vi "UWB_Controller.vi"() -> ()   [LabVIEW 2016]
doc: "This VI controlls the DWM over UART. It starts of by resetting the DWM by sending a reset message over UART. It then starts sending CR messages to the DWM and poll for a response. When anything is received on the poll the DWM is operational. It then starts to request a position message which it saves in a global variable later used by the ROS publisher."
uses:
  <vilib>/myRIO/Instrument Drivers/Onboard IO/AO/typedefs/AO Reference.ctl
  <vilib>/myRIO/Common/Instrument Driver Framework/Utilities/typedefs/myRIO Generic Hardware Reference.ctl
  <vilib>/myRIO/Common/Instrument Driver Framework/Utilities/typedefs/Hardware Version Enum.ctl
  <vilib>/myRIO/Common/Instrument Driver Framework/Utilities/typedefs/myRIO v1.0 Reference.ctl
  <vilib>/myRIO/Common/Instrument Driver Framework/Utilities/typedefs/Generic FPGA Reference.ctl
  <vilib>/myRIO/Common/Instrument Driver Framework/myRIO v1.0/AO/typedefs/AO Channels List.ctl
  <vilib>/myRIO/Common/Instrument Driver Framework/myRIO v1.0/AO/typedefs/AO Channels Enum.ctl
  <vilib>/myRIO/Common/Instrument Driver Framework/Utilities/typedefs/Analog Scaling Constants List.ctl
  <vilib>/myRIO/Common/Instrument Driver Framework/Utilities/typedefs/Analog Scaling Constants.ctl
  <vilib>/userdefined/High Color/nirio_resource_hc.ctl
  <vilib>/myRIO/Instrument Drivers/Onboard IO/UART/typedef/VISA Configuration.ctl
  <vilib>/myRIO/Instrument Drivers/Onboard IO/DIO/typedefs/DIO Reference.ctl
  <vilib>/myRIO/Common/Instrument Driver Framework/myRIO v1.0/DIO/typedefs/DIO Channels List.ctl
  <vilib>/myRIO/Common/Instrument Driver Framework/myRIO v1.0/DIO/typedefs/DIO Channels Enum.ctl
  <vilib>/myRIO/Common/Instrument Driver Framework/Utilities/vis/Is FPGA Ref Available.vi
  <vilib>/myRIO/Common/Instrument Driver Framework/roboRIO v1.0/AO/vis/roboRIO v1.0 Open AO.vi
  <vilib>/myRIO/Instrument Drivers/Onboard IO/AO/vis/Write.vi
  <vilib>/myRIO/Common/Instrument Driver Framework/roboRIO v1.0/DIO/vis/roboRIO v1.0 Open DIO.vi
  <vilib>/myRIO/Instrument Drivers/Onboard IO/DIO/vis/Write.vi
  <vilib>/myRIO/Common/Instrument Driver Framework/Utilities/vis/Validate Channels.vi
  <vilib>/myRIO/Common/Instrument Driver Framework/roboRIO v1.0/AO/vis/roboRIO v1.0 Reserve AO.vi
  <vilib>/myRIO/Common/Instrument Driver Framework/roboRIO v1.0/DIO/vis/roboRIO v1.0 Reserve DIO.vi
  <vilib>/myRIO/Common/Instrument Driver Framework/roboRIO v1.0/AO/vis/roboRIO v1.0 Build MUX Configuration AO.vi
  <vilib>/myRIO/Common/Instrument Driver Framework/roboRIO v1.0/Resource Manager/vis/roboRIO v1.0 Reserve Channel List.vi
  <vilib>/myRIO/Common/Instrument Driver Framework/roboRIO v1.0/DIO/vis/roboRIO v1.0 Build MUX Configuration DIO.vi
  <vilib>/myRIO/Common/Instrument Driver Framework/roboRIO v1.0/Resource Manager/vis/roboRIO v1.0 Reserve Channel.vi
  <vilib>/myRIO/Common/Instrument Driver Framework/roboRIO v1.0/Resource Manager/vis/roboRIO v1.0 Unreserve Channel.vi
  <vilib>/myRIO/Common/Instrument Driver Framework/roboRIO v1.0/Resource Manager/vis/roboRIO v1.0 Create Configuration List.vi
  <vilib>/myRIO/Common/Instrument Driver Framework/roboRIO v1.0/Resource Manager/vis/roboRIO v1.0 Build Mutex Name.vi
  <vilib>/Instr/_visa.llb/VISA Configure Serial Port (Instr).vi
  GlobalVI.vi
  <vilib>/Utility/VariantDataType/GetNumericInfo.vi
  <vilib>/Utility/error.llb/Error Cluster From Error Code.vi
  <vilib>/myRIO/Common/Instrument Driver Framework/roboRIO v1.0/roboRIO v1.0 Open.vi
  <vilib>/myRIO/Common/Instrument Driver Framework/Utilities/vis/IO Manager.vi
  <vilib>/myRIO/Common/Instrument Driver Framework/Utilities/vis/Configuration Manager.vi
  <vilib>/myRIO/Common/Instrument Driver Framework/roboRIO v1.0/Resource Manager/vis/roboRIO v1.0 Configure IO.vi
  <vilib>/myRIO/Common/Instrument Driver Framework/myRIO v1.0/myRIO v1.0 Close.vi
  <vilib>/myRIO/Common/Instrument Driver Framework/roboRIO v1.0/DIO/vis/roboRIO v1.0 Write DIO.vi
  <vilib>/myRIO/Common/Instrument Driver Framework/roboRIO v1.0/AO/vis/roboRIO v1.0 Get Scaling Constants AO.vi
  <vilib>/myRIO/Common/Instrument Driver Framework/roboRIO v1.0/AO/vis/roboRIO v1.0 Write AO.vi
  <vilib>/myRIO/Express VI/Onboard IO/UART/UART Express VI.xnode
  <vilib>/regexp/Match Regular Expression.xnode
  <vilib>/myRIO/Express VI/Onboard Devices/LED/LED Express VI.xnode
  <vilib>/myRIO/Instrument Drivers/Onboard IO/DIO/vis/myRIO DIO Open.xnode
  <vilib>/myRIO/Express VI/Onboard IO/AO/AO Express VI.xnode
  <vilib>/myRIO/Instrument Drivers/Onboard IO/AO/vis/myRIO AO Open.xnode
  <vilib>/myRIO/Instrument Drivers/Onboard IO/UART/UART.lvlib
  <vilib>/myRIO/Instrument Drivers/Onboard IO/DIO/DIO.lvlib
  <vilib>/myRIO/Instrument Drivers/Onboard IO/AO/AO.lvlib
panel:
  in  "error in OUTPUT 3":errorcluster
  in  "error in INPUT 2":errorcluster
  out "currentTimeout_Receive":u32
  out "error out OUTPUT 2":errorcluster
  out "offset past match\n(-1 = no match)":i32
  out "MSGFound":bool
  out "X":dbl
  out "Y":dbl
  out "Z":dbl
  out "error out INPUT":errorcluster
  out "timeoutError":bool
  out "currentTimeout":u32
  out "timeoutCount":u32
  out "timeoutValue":u32
  out "Resetting...":bool
  out "System ON":bool
  out "Receiving":bool
  out "Transmitting":bool
  out "UART Reset Buffer":string
  out "uwbState":i32
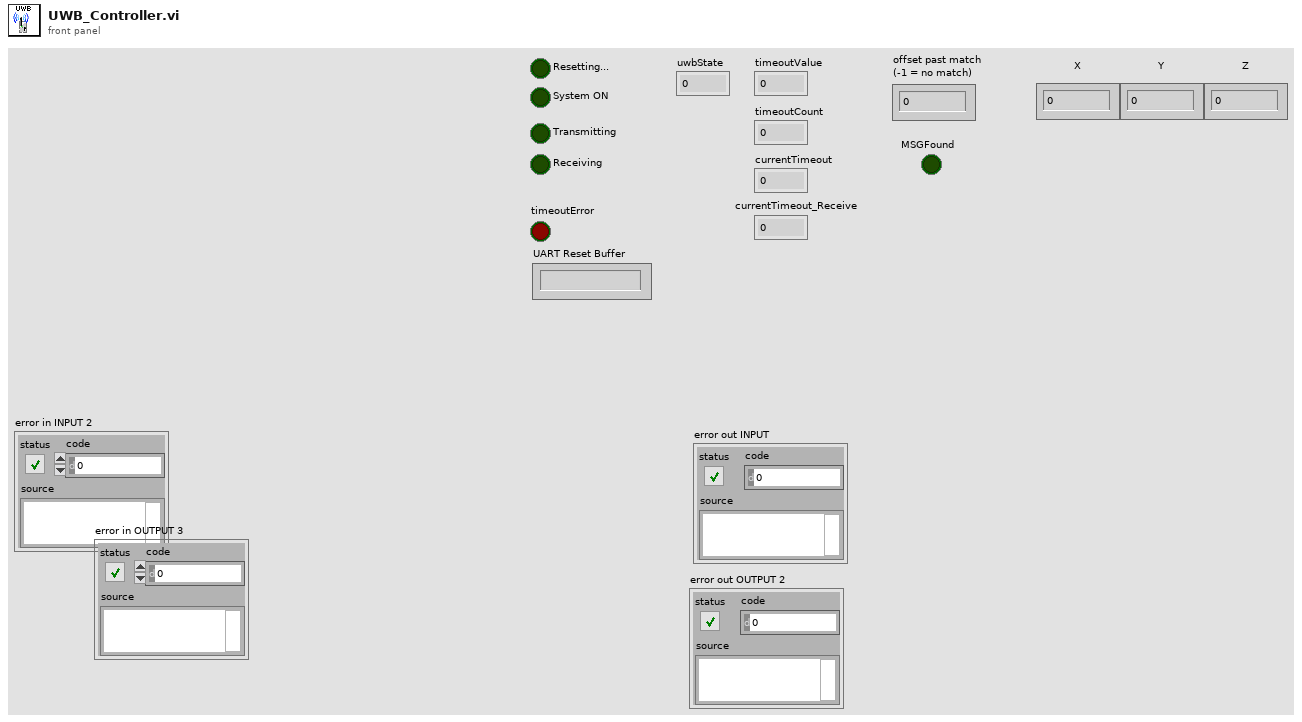
[diagram p1: front panel]
types:
  T1 = typedef "UART.lvlib/VISA Configuration.ctl" = cluster{"baud rate (9600)":u32, "data bits (8)":u16, "parity (0:none)":enum16{"None", "Odd", "Even", "Mark", "Space"}, "stop bits (10: 1 bit)":u16, "flow control (0:none)":u16, "termination char\n(0xA = '\\n' = LF) ":u8, "Enable Termination\nChar (T)":bool, "timeout (10sec)":u32}
  T2 = typedef "DIO.lvlib/DIO Reference.ctl" = cluster{"myRIO Reference":T3, "DIO Channels List":T7}
  T3 = typedef "myRIO Generic Hardware Reference.ctl" = cluster{"myRIO Model":T4, "myRIO Hardware Reference":T5}
  T4 = typedef "Hardware Version Enum.ctl" = enum16{"Unknown", "myRIO-1900", "myRIO-1950", "roboRIO", "NI ELVIS RIO CM"}
  T5 = typedef "myRIO v1.0 Reference.ctl" = cluster{"Generic FPGA Reference":T6, "Allow multiple opens":bool}
  T6 = typedef "Generic FPGA Reference.ctl" = refnum<k20>
  T7 = typedef "DIO Channels List.ctl" = T8[]
  T8 = typedef "DIO Channels Enum.ctl" = enum16{"Not Connected", "C/DIO0", "C/DIO1", "C/DIO2", "C/DIO3", "C/DIO4", "C/DIO5", "C/DIO6", "C/DIO7", "A/DIO0", "A/DIO1", "A/DIO2", "A/DIO3", "A/DIO4", "A/DIO5", "A/DIO6", "A/DIO7", "A/DIO8", "A/DIO9", "A/DIO10", "A/DIO11", "A/DIO12", "A/DIO13", "A/DIO14", "A/DIO15", "B/DIO0", "B/DIO1", "B/DIO2", "B/DIO3", "B/DIO4", "B/DIO5", "B/DIO6", "B/DIO7", "B/DIO8", "B/DIO9", "B/DIO10", "B/DIO11", "B/DIO12", "B/DIO13", "B/DIO14", "B/DIO15", "LED0", "LED1", "LED2", "LED3", "Button0", "DIO/DIO0", "DIO/DIO1", "DIO/DIO2", "DIO/DIO3", "DIO/DIO4", "DIO/DIO5", "DIO/DIO6", "DIO/DIO7", "DIO/DIO8", "DIO/DIO9", "SPI/CS0", "SPI/CS1", "SPI/CS2", "SPI/CS3", "LED RADIO (Green)", "LED RADIO (Red)", "LED COMM (Green)", "LED COMM (Red)", "LED MODE (Green)", "LED MODE (Red)"}
  T9 = typedef "nirio_resource_hc.ctl" = tag
  T10 = typedef "AO.lvlib/AO Reference.ctl" = cluster{"myRIO Reference":T3, "AO Channel List":T11, "AO Scaling Constant List":T13}
  T11 = typedef "AO Channels List.ctl" = T12[]
  T12 = typedef "AO Channels Enum.ctl" = enum16{"Not Connected", "AudioOut/Left", "AudioOut/Right", "C/AO0", "C/AO1", "A/AO0", "A/AO1", "B/AO0", "B/AO1"}
  T13 = typedef "Analog Scaling Constants List.ctl" = T14[]
  T14 = typedef "Analog Scaling Constants.ctl" = cluster{"LSB Weight (Volts)":dbl, "Offset (Volts)":dbl, "Signed?":bool}
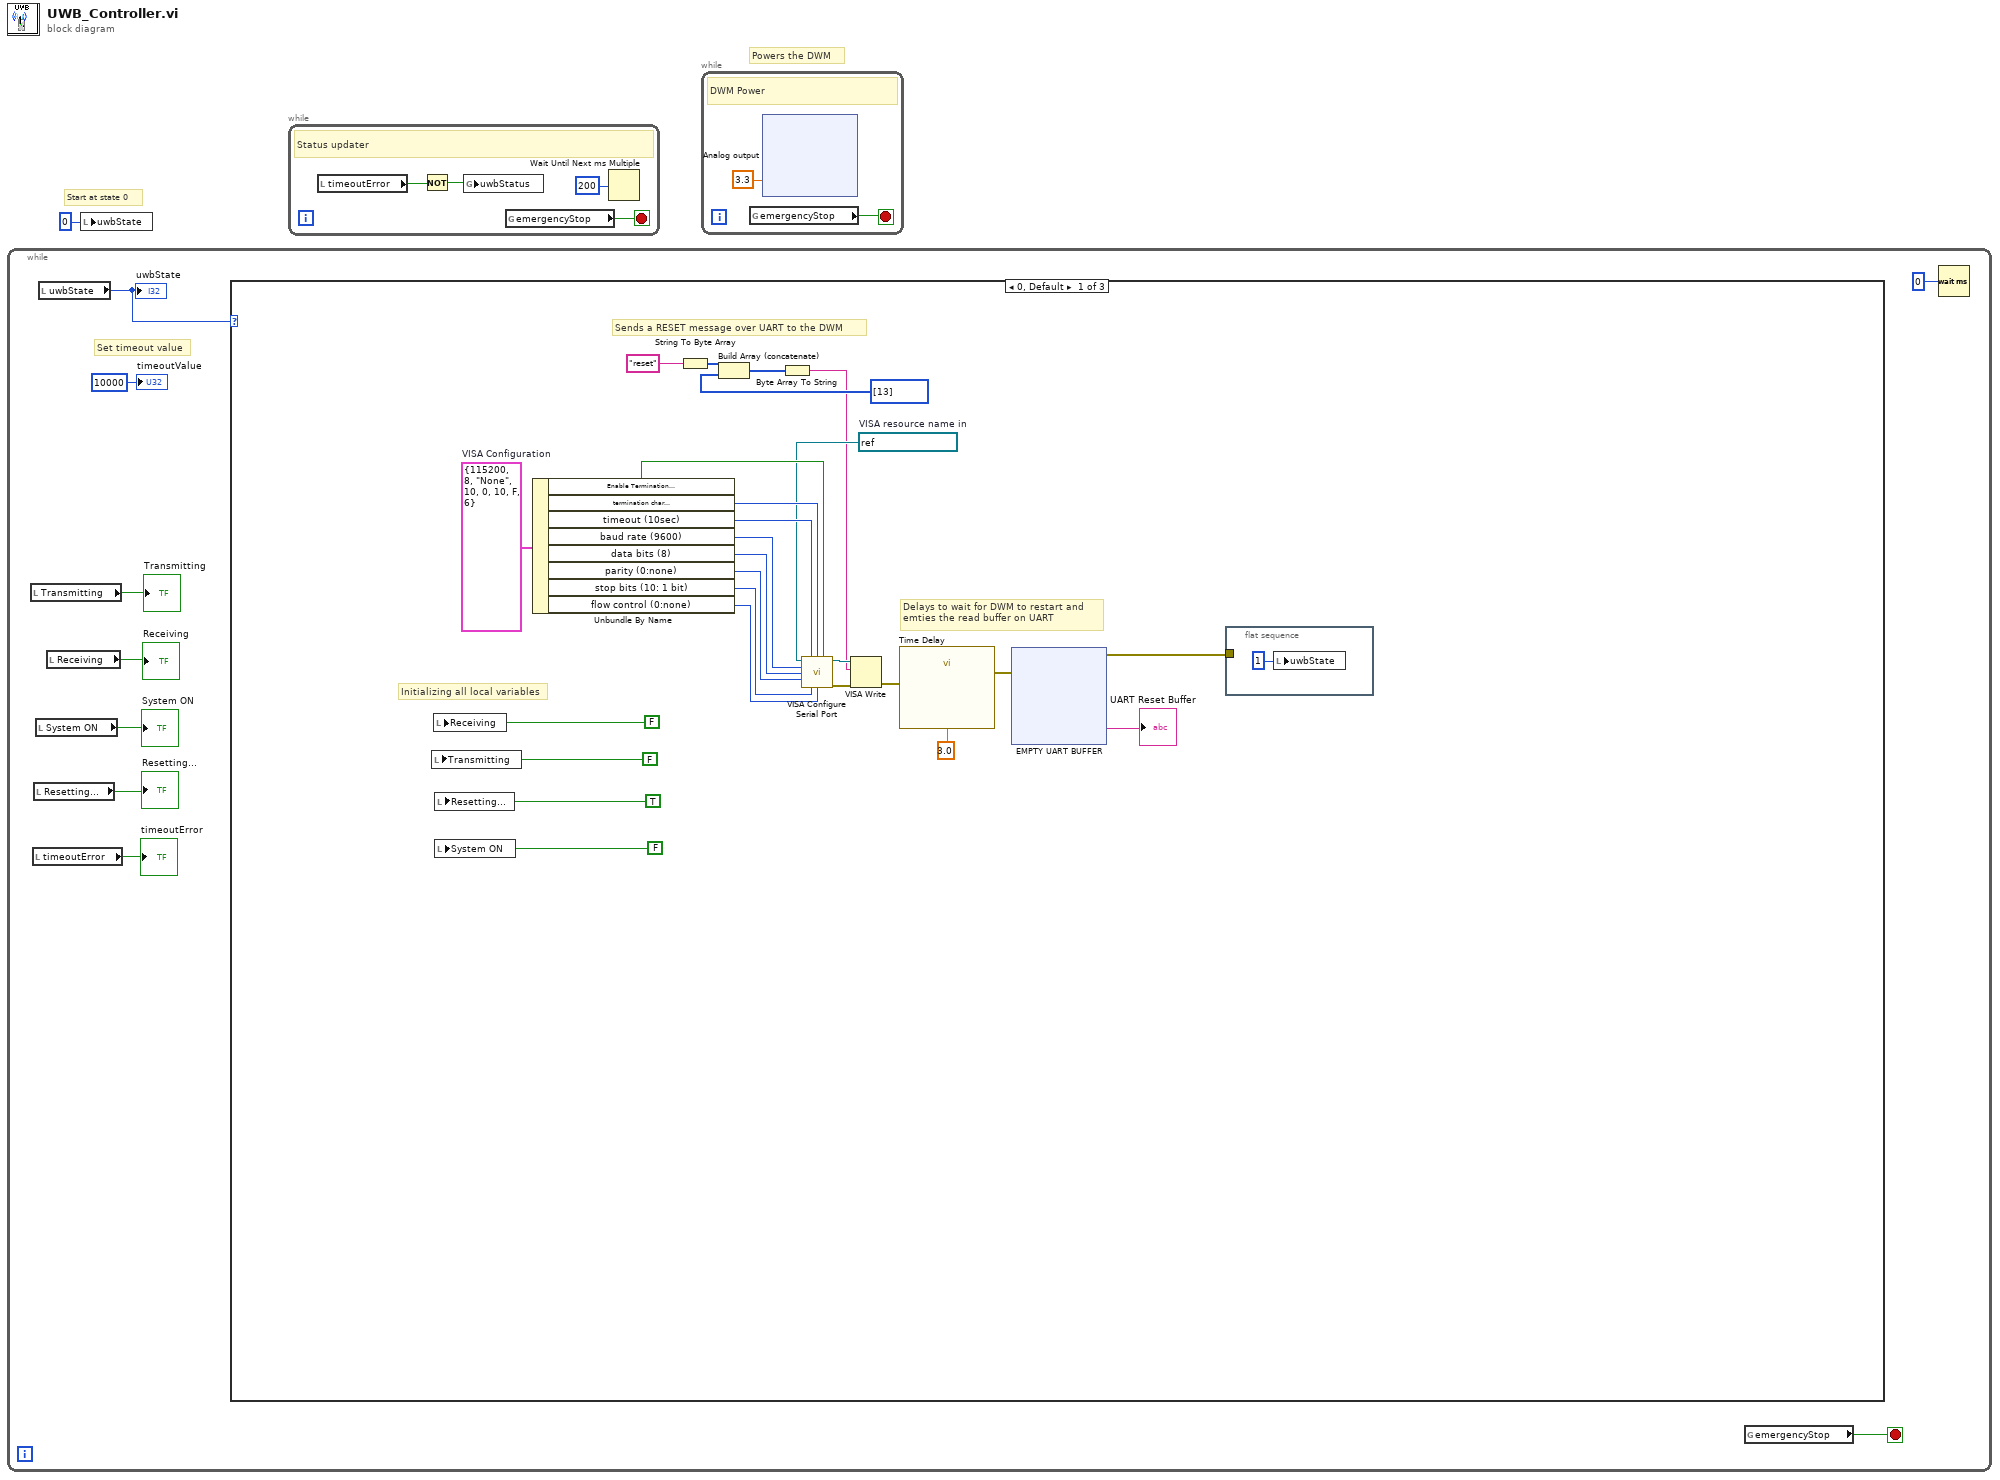
[diagram p0: block diagram]
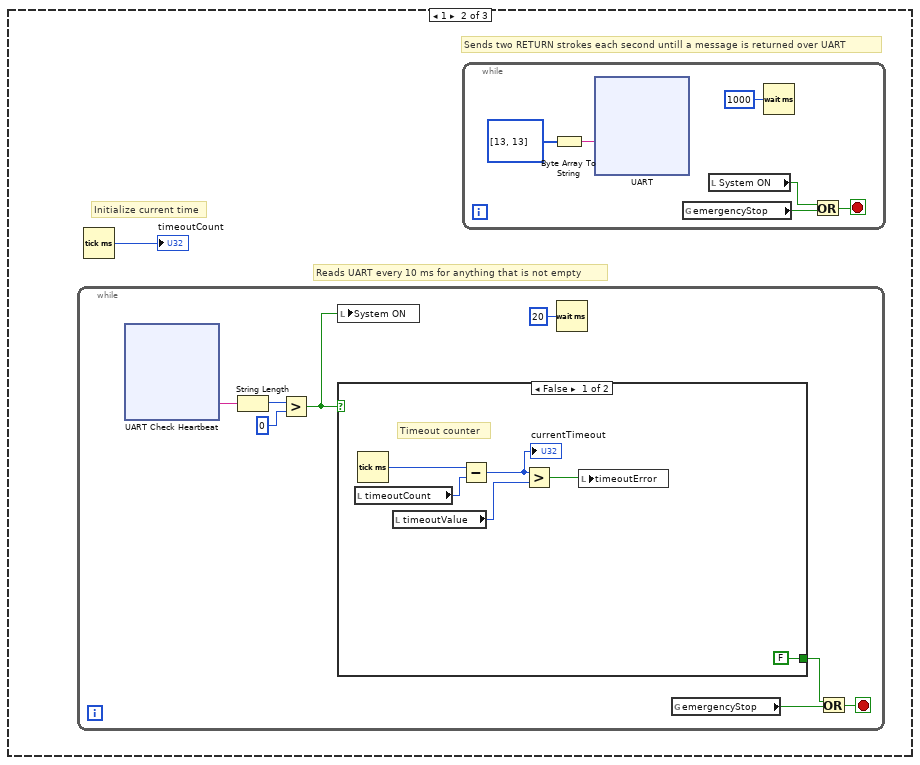
[diagram p2: hidden frame]
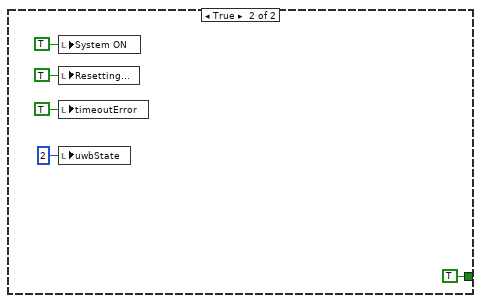
[diagram p3: hidden frame]
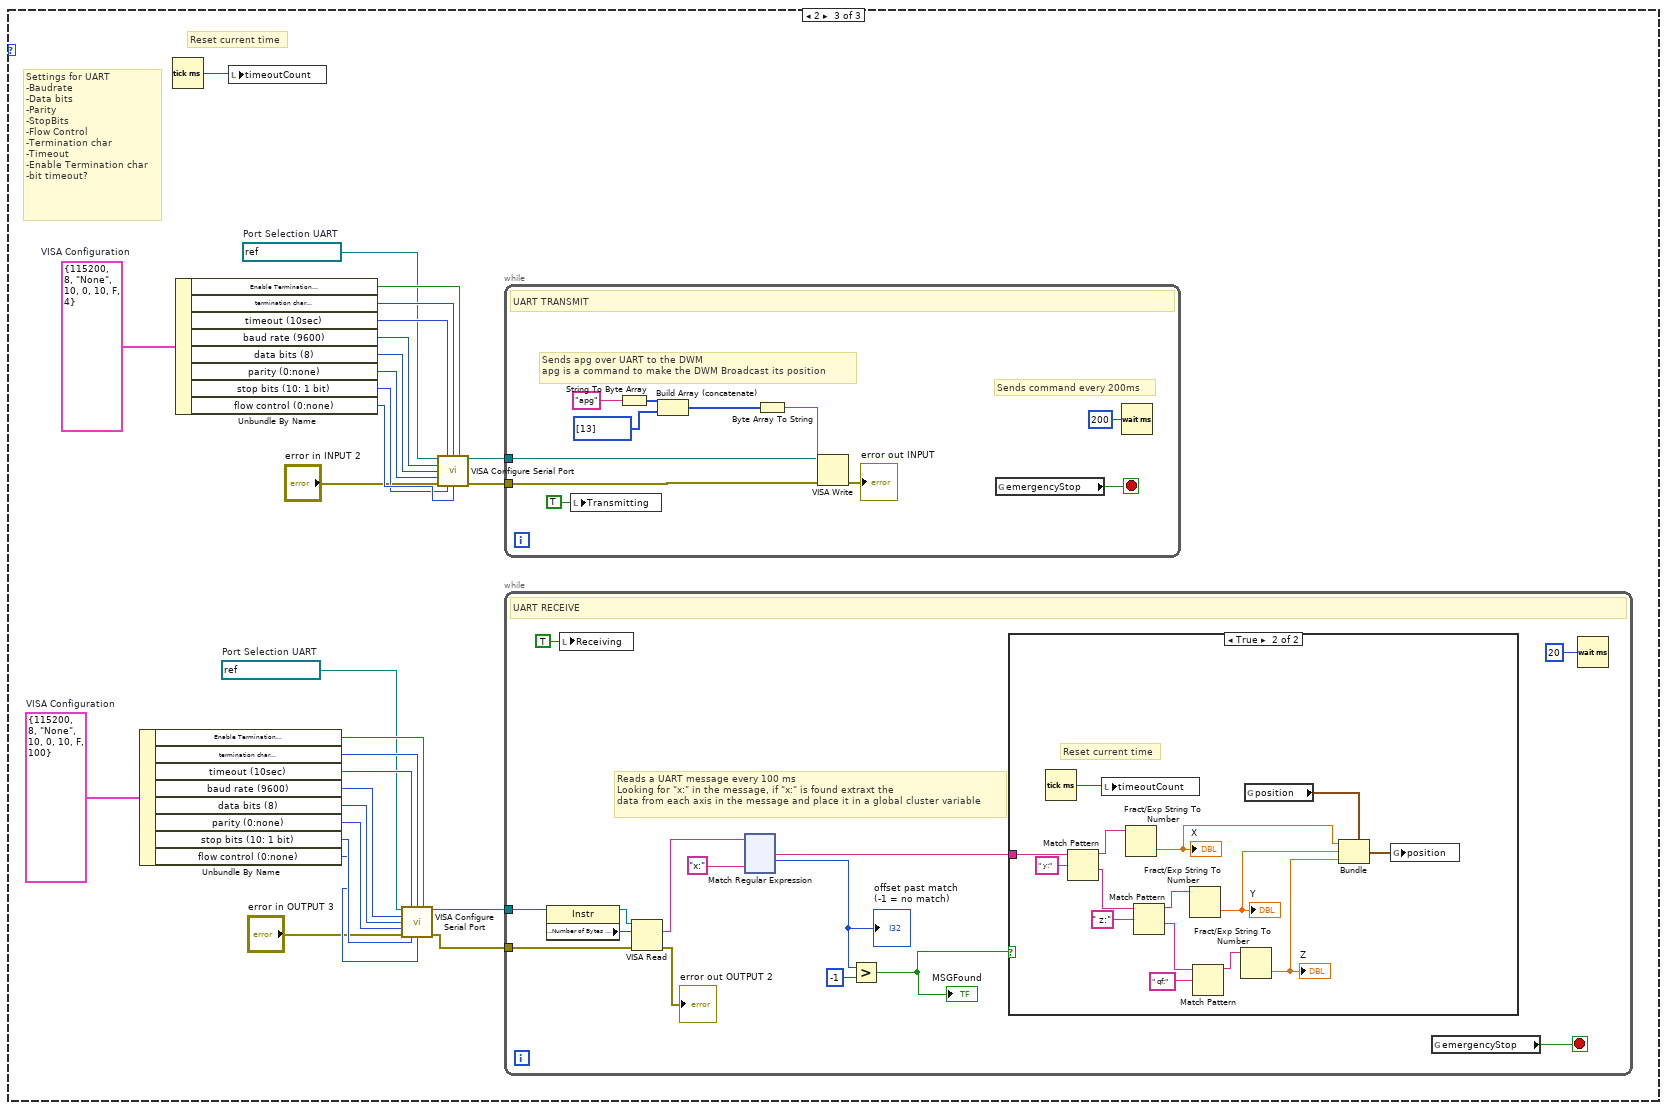
[diagram p4: hidden frame]
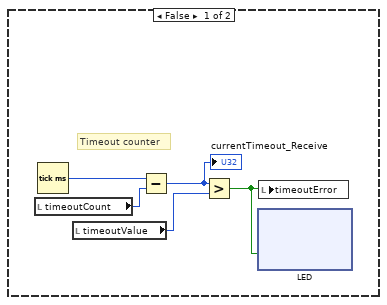
[diagram p5: hidden frame]
diagram:
  # "Powers the DWM"
  # "Start at state 0"
  n1 = while {
    stop <- w6 stop-if-true
    # "Set timeout value"
    n2 = local read "Transmitting"() -> (→"Transmitting":bool)
    n3 = local read "timeoutError"() -> (→"timeoutError":bool)
    n4 = local read "Resetting..."() -> (→"Resetting...":bool)
    n5 = local read "System ON"() -> (→"System ON":bool)
    n6 = local read "uwbState"() -> (w4:i32)
    "uwbState" <- w4
    n7 = local read "Receiving"() -> (→"Receiving":bool)
    n8 = case shown="0, Default" w4 {
      frame 0, Default {
        w24 = T1 {"baud rate (9600)"=115200, "data bits (8)"=8, "parity (0:none)"=enum."None", "stop bits (10: 1 bit)"=10, "flow control (0:none)"=0, "termination char\n(0xA = '\\n' = LF) "=10, "Enable Termination\nChar (T)"=FALSE, "timeout (10sec)"=6}  # VISA Configuration
        w23 = refnum<visa-resource-name> "ASRL2::INSTR"  # VISA resource name in
        # "Initializing all local variables"
        # "Delays to wait for DWM to restart and \nemties the read buffer on UART"
        # "Sends a RESET message over UART to the DWM"
        n9 = local write "Transmitting"(FALSE ("Transmitting")) -> ()
        n10 = local write "Receiving"(FALSE ("Receiving")) -> ()
        n11 = local write "Resetting..."(TRUE ("Resetting...")) -> ()
        n12 = local write "System ON"(FALSE ("System On")) -> ()
        n13 = Unbundle By Name(w24) -> ("Enable Termination\nChar (T)"=w27:bool, "termination char\n(0xA = '\\n' = LF)"=w28:u8, "timeout (10sec)"=w29:u32, "baud rate (9600)"=w34:u32, "data bits (8)"=w33:u16, "parity (0:none)"=w32:enum16{"None", "Odd", "Even", "Mark", "Space"}, "stop bits (10: 1 bit)"=w31:u16, "flow control (0:none)"=w30:u16)
        n14 = String To Byte Array(string="reset") -> (unsigned byte array=w19:u8[])
        n15 = Build Array (concatenate)(w19, i32[] [13]) -> (w18:i32[])
        n16 = Byte Array To String(unsigned byte array=w18) -> (string=w17:string)
        n17 = call-poly "VISA Configure Serial Port"("VISA resource name"=w23, "timeout (10sec)"=w29, "termination char\n(0xA = '\\n' = LF)"=w28, "Enable Termination\nChar (T)"=w27, "baud rate (9600)"=w34, "data bits (8)"=w33, "parity (0:none)"=w32, "stop bits (10: 1 bit)"=w31, "flow control (0:none)"=w30) -> ("VISA resource name out"=w25:refnum<visa-resource-name>, "error out"=w26:errorcluster)  [unwired: 5 in]
        n18 = VISA Write(VISA resource name=w25, write buffer=w17, error in (no error)=w26) -> (error out=w22:errorcluster)  [unwired: 2 out]
        n19 = call "Time Delay"("error in (no error)"=w22, "Delay Time (s)"=3.0) -> ("error out"=w35:errorcluster)  [unwired: 9 in]
        n20 = xnode "EMPTY UART BUFFER"("error in (no error)"=w35) -> ("Characters Read"=→"UART Reset Buffer":string, "error out"=w11:errorcluster)
        n21 = flat-sequence {
          tunnel: w11 -> [_]
          frame #0 {
            n22 = local write "uwbState"(1 ("uwbState")) -> ()
          }
        }
      }
      frame 1 {
        # "Initialize current time"
        # "Reads UART every 10 ms for anything that is not empty"
        # "Sends two RETURN strokes each second untill a message is returned over UART"
        n23 = while {
          stop <- w80 stop-if-true
          n24 = xnode "UART Check Heartbeat"() -> ("Characters Read"=w85:string)  [unwired: 1 in, 1 out]
          n25 = String Length(string=w85) -> (length=w84:i32)
          n26 = Greater?(x=w84, y=0) -> (0:w81:bool)
          n27 = local write "System ON"(w81) -> ()
          n28 = case shown="False" w81 {
            tunnel: [FALSE TRUE] -> w79
            frame False {
              # "Timeout counter"
              n29 = local read "timeoutCount"() -> (w88:u32)
              n30 = Tick Count (ms)() -> (millisecond timer value=w90:u32)
              n31 = local read "timeoutValue"() -> (w89:u32)
              n32 = Subtract(x=w90, y=w88) -> (x-y=w87:u32)
              "currentTimeout" <- w87
              n33 = Greater?(x=w87, y=w89) -> (0:w86:bool)
              n34 = local write "timeoutError"(w86) -> ()
            }
            frame True {
              n35 = local write "System ON"(TRUE ("System ON")) -> ()
              n36 = local write "Resetting..."(TRUE ("Resetting...")) -> ()
              n37 = local write "timeoutError"(TRUE ("timeoutError")) -> ()
              n38 = local write "uwbState"(2 ("uwbState")) -> ()
            }
          }
          n39 = Wait (ms)(milliseconds to wait=u32 20) -> ()  [unwired: 1 out]
          n40 = global read "GlobalVI.vi" "emergencyStop"() -> (w78:bool)
          n41 = Or(x=w79, y=w78) -> (x .or. y?=w80:bool)
        }
        n42 = Tick Count (ms)() -> (millisecond timer value=→"timeoutCount":u32)
        n43 = while {
          stop <- w57 stop-if-true
          n44 = Byte Array To String(unsigned byte array=u8[] [13, 13]) -> (string=w61:string)
          n45 = xnode "UART"("Characters to Write"=w61) -> ()  [unwired: 1 in, 2 out]
          n46 = global read "GlobalVI.vi" "emergencyStop"() -> (w58:bool)
          n47 = local read "System ON"() -> (w56:bool)
          n48 = Wait (ms)(milliseconds to wait=u32 1000) -> ()  [unwired: 1 out]
          n49 = Or(x=w56, y=w58) -> (x .or. y?=w57:bool)
        }
      }
      frame 2 {
        w117 = T1 {"baud rate (9600)"=115200, "data bits (8)"=8, "parity (0:none)"=enum."None", "stop bits (10: 1 bit)"=10, "flow control (0:none)"=0, "termination char\n(0xA = '\\n' = LF) "=10, "Enable Termination\nChar (T)"=FALSE, "timeout (10sec)"=100}  # VISA Configuration
        w116 = refnum<visa-resource-name> "ASRL2::INSTR"  # Port Selection UART
        w130 = T1 {"baud rate (9600)"=115200, "data bits (8)"=8, "parity (0:none)"=enum."None", "stop bits (10: 1 bit)"=10, "flow control (0:none)"=0, "termination char\n(0xA = '\\n' = LF) "=10, "Enable Termination\nChar (T)"=FALSE, "timeout (10sec)"=4}  # VISA Configuration
        w129 = refnum<visa-resource-name> "ASRL2::INSTR"  # Port Selection UART
        # "Settings for UART\n-Baudrate\n-Data bits\n-Parity\n-StopBits\n-Flow Control\n-Termination char\n-Timeout\n-Enable Termination char\n-bit timeout?"
        # "Reset current time"
        n50 = Unbundle By Name(w117) -> ("Enable Termination\nChar (T)"=w119:bool, "termination char\n(0xA = '\\n' = LF)"=w120:u8, "timeout (10sec)"=w121:u32, "baud rate (9600)"=w126:u32, "data bits (8)"=w125:u16, "parity (0:none)"=w124:enum16{"None", "Odd", "Even", "Mark", "Space"}, "stop bits (10: 1 bit)"=w123:u16, "flow control (0:none)"=w122:u16)
        n51 = Tick Count (ms)() -> (millisecond timer value=w140:u32)
        n52 = Unbundle By Name(w130) -> ("Enable Termination\nChar (T)"=w132:bool, "termination char\n(0xA = '\\n' = LF)"=w133:u8, "timeout (10sec)"=w134:u32, "baud rate (9600)"=w138:u32, "data bits (8)"=w137:u16, "parity (0:none)"=w136:enum16{"None", "Odd", "Even", "Mark", "Space"}, "stop bits (10: 1 bit)"=w135:u16, "flow control (0:none)"=w139:u16)
        n53 = local write "timeoutCount"(w140) -> ()
        n54 = call-poly "VISA Configure Serial Port"("VISA resource name"=w116, "timeout (10sec)"=w121, "termination char\n(0xA = '\\n' = LF)"=w120, "Enable Termination\nChar (T)"=w119, "baud rate (9600)"=w126, "data bits (8)"=w125, "parity (0:none)"=w124, "error in (no error)"="error in OUTPUT 3", "stop bits (10: 1 bit)"=w123, "flow control (0:none)"=w122) -> ("VISA resource name out"=w115:refnum<visa-resource-name>, "error out"=w114:errorcluster)  [unwired: 4 in]
        n55 = call-poly "VISA Configure Serial Port"("VISA resource name"=w129, "timeout (10sec)"=w134, "termination char\n(0xA = '\\n' = LF)"=w133, "Enable Termination\nChar (T)"=w132, "baud rate (9600)"=w138, "data bits (8)"=w137, "parity (0:none)"=w136, "error in (no error)"="error in INPUT 2", "stop bits (10: 1 bit)"=w135, "flow control (0:none)"=w139) -> ("VISA resource name out"=w128:refnum<visa-resource-name>, "error out"=w127:errorcluster)  [unwired: 4 in]
        n56 = while {
          tunnel: w128 -> [w325]
          tunnel: w127 -> [w324]
          stop <- w326 stop-if-true
          # "Sends command every 200ms"
          # "Sends apg over UART to the DWM\napg is a command to make the DWM Broadcast its position"
          # "UART TRANSMIT"
          n57 = local write "Transmitting"(TRUE ("Transmitting")) -> ()
          n58 = String To Byte Array(string="apg") -> (unsigned byte array=w331:u8[])
          n59 = Build Array (concatenate)(w331, i32[] [13]) -> (w330:i32[])
          n60 = Byte Array To String(unsigned byte array=w330) -> (string=w334:string)
          n61 = VISA Write(VISA resource name=w325, write buffer=w334, error in (no error)=w324) -> (error out=→"error out INPUT":errorcluster)  [unwired: 2 out]
          n62 = global read "GlobalVI.vi" "emergencyStop"() -> (w326:bool)
          n63 = Wait (ms)(milliseconds to wait=u32 200) -> ()  [unwired: 1 out]
        }
        n64 = while {
          tunnel: w115 -> [w142]
          tunnel: w114 -> [w141]
          stop <- w143 stop-if-true
          # "Reads a UART message every 100 ms\nLooking for \"x:\" in the message, if \"x:\" is found extraxt the\ndata from each axis in the message and place it in a global cluster variable"
          # "UART RECEIVE"
          n65 = property class="Instr"(reference=w142) -> (reference out=w152:refnum<visa-resource-name>, "Serial Settings:Number of Bytes at Serial Port"=w153:u32)  [unwired: 1 in, 1 out]
          n66 = local write "Receiving"(TRUE ("Receiving")) -> ()
          n67 = VISA Read(VISA resource name=w152, byte count=w153, error in (no error)=w141) -> (read buffer=w146:string, error out=→"error out OUTPUT 2":errorcluster)  [unwired: 2 out]
          n68 = xnode "Match Regular Expression"("input string"=w146, "regular expression"="x:") -> ("after match"=w145:string, "offset past match"=w149:i32)  [unwired: 4 in, 3 out]
          "offset past match\n(-1 = no match)" <- w149
          n69 = Greater?(x=w149, y=-1) -> (0:w147:bool)
          "MSGFound" <- w147
          n70 = case shown="True" w147 {
            tunnel: w145 -> [_ w201]
            frame False {
              # "Timeout counter"
              n71 = local read "timeoutCount"() -> (w157:u32)
              n72 = Tick Count (ms)() -> (millisecond timer value=w159:u32)
              n73 = local read "timeoutValue"() -> (w158:u32)
              n74 = Subtract(x=w159, y=w157) -> (x-y=w156:u32)
              "currentTimeout_Receive" <- w156
              n75 = Greater?(x=w156, y=w158) -> (0:w155:bool)
              n76 = xnode "LED"("RADIO (Red)"=w155) -> ()  [unwired: 1 in, 1 out]
              n77 = local write "timeoutError"(w155) -> ()
            }
            frame True {
              # "Reset current time"
              n78 = Tick Count (ms)() -> (millisecond timer value=w196:u32)
              n79 = Match Pattern(string=w201, regular expression=" y:") -> (before substring=w208:string, after substring=w207:string)  [unwired: 1 in, 2 out]
              n80 = local write "timeoutCount"(w196) -> ()
              n81 = Fract/Exp String To Number(string=w208) -> (number=w199:dbl)  [unwired: 3 in, 1 out]
              "X" <- w199
              n82 = Match Pattern(string=w207, regular expression=" z:") -> (before substring=w205:string, after substring=w206:string)  [unwired: 1 in, 2 out]
              n83 = Fract/Exp String To Number(string=w205) -> (number=w198:dbl)  [unwired: 3 in, 1 out]
              "Y" <- w198
              n84 = Match Pattern(string=w206, regular expression=" qf:") -> (before substring=w204:string)  [unwired: 1 in, 3 out]
              n85 = Fract/Exp String To Number(string=w204) -> (number=w197:dbl)  [unwired: 3 in, 1 out]
              "Z" <- w197
              n86 = global read "GlobalVI.vi" "position"() -> (w200:cluster{"x":dbl, "y":dbl, "z":dbl})
              n87 = Bundle(cluster=w200, "x"=w199, "y"=w198, "z"=w197) -> (w195:cluster{"x":dbl, "y":dbl, "z":dbl})
              n88 = global write "GlobalVI.vi" "position"(w195) -> ()
            }
          }
          n89 = global read "GlobalVI.vi" "emergencyStop"() -> (w143:bool)
          n90 = Wait (ms)(milliseconds to wait=u32 20) -> ()  [unwired: 1 out]
        }
      }
    }
    n91 = global read "GlobalVI.vi" "emergencyStop"() -> (w6:bool)
    n92 = Wait (ms)(milliseconds to wait=u32 0) -> ()  [unwired: 1 out]
    "timeoutValue" <- u32 10000 ("timeoutValue")
  }
  n93 = local write "uwbState"(0 ("uwbState")) -> ()
  n94 = while {
    stop <- w338 stop-if-true
    # "Status updater"
    n95 = local read "timeoutError"() -> (w337:bool)
    n96 = Not(x=w337) -> (.not. x?=w336:bool)
    n97 = global write "GlobalVI.vi" "uwbStatus"(w336) -> ()
    n98 = global read "GlobalVI.vi" "emergencyStop"() -> (w338:bool)
    n99 = Wait Until Next ms Multiple(millisecond multiple=u32 200) -> ()  [unwired: 1 out]
  }
  n100 = while {
    stop <- w340 stop-if-true
    # "DWM Power"
    n101 = global read "GlobalVI.vi" "emergencyStop"() -> (w340:bool)
    n102 = xnode "Analog output"("B/AO1 (Pin 4)"=3.3) -> ()  [unwired: 1 in, 1 out]
  }
